vi "SD Write Num Rarely.vi"(6 "Iterations":i32=10, 9 "Numeric":dbl, 11 "Name":string="Numeric") -> ()   [LabVIEW 2013]
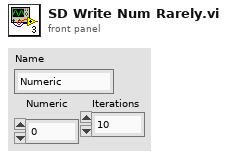
[diagram p1: front panel]
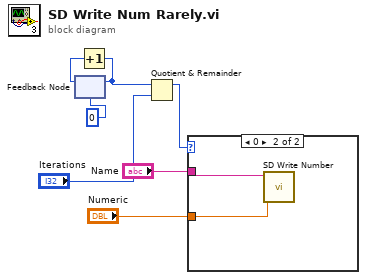
[diagram p0: block diagram]
diagram:
  n1 = feedback #1(0) -> (w4:i32)
  n2 = Increment(x=w4) -> (x+1=w3:i32)
  n3 = feedback-in #1(w3) -> ()
  n4 = Quotient & Remainder(x=w3, y="Iterations") -> (x-y*floor(x/y)=w1:i32)  [unwired: 1 out]
  n5 = case shown="0" w1 {
    tunnel: "Name" -> [_ w9]
    tunnel: "Numeric" -> [_ w8]
    frame Default {
    }
    frame 0 {
      n6 = call <vilib>:"SD Write Number.vi"("Numeric"=w8, "Name"=w9) -> ()  [unwired: 8 in, 2 out]
    }
  }
